vi "NM GlobalTest.vi"() -> ()   [LabVIEW 2010] (continued)
                        }
                        frame "DAQmx" {
                          n691 = call-poly <vilib>:"DAQmx Read.vi"("task/channels in"=w2908, "number of samples per channel"=w2904, "timeout"=w2905, "error in"=w2909) -> ("task out"=w2911:refnum<k21>, "data"=w2906:dbl[], "error out"=w2910:errorcluster)  [unwired: 9 in]
                        }
                      }
                      "data 37" <- w2890
                      "data 75" <- w2890
                    }
                    frame "sCnSWfm" {
                      n692 = case shown="\"DAQmx\"" w2914 {
                        tunnel: [w2927 w2935] -> w2921
                        tunnel: [w2928 w2932] -> w2920
                        tunnel: [w2929 w2937] -> w2915
                        tunnel: w2919 -> [w2925 w2933]
                        tunnel: w2918 -> [w2926 w2932]
                        tunnel: [w2924 w2936] -> w2917
                        tunnel: w2916 -> [w2924 w2934]
                        tunnel: w2913 -> [w2923 w2931]
                        tunnel: "samples per" -> [w2922 w2930]
                        frame "ULx", Default {
                          n693 = call-poly <vilib>:"ULx Read.vi"("task in"=w2926, "number of samples per channel"=w2922, "timeout"=w2923, "error in"=w2925) -> ("task out"=w2928:refnum<k24>, "data"=w2929:waveform(dbl), "error out"=w2927:errorcluster)  [unwired: 9 in]
                        }
                        frame "DAQmx" {
                          n694 = call-poly <vilib>:"DAQmx Read.vi"("task/channels in"=w2934, "number of samples per channel"=w2930, "timeout"=w2931, "error in"=w2933) -> ("task out"=w2936:refnum<k21>, "data"=w2937:waveform(dbl), "error out"=w2935:errorcluster)  [unwired: 9 in]
                        }
                      }
                      "data 38" <- w2915
                    }
                    frame "nCsSDbl" {
                      n695 = case shown="\"DAQmx\"" w2939 {
                        tunnel: [w2952 w2955] -> w2946
                        tunnel: [w2951 w2958] -> w2945
                        tunnel: [w2953 w2960] -> w2940
                        tunnel: w2944 -> [w2950 w2957]
                        tunnel: w2943 -> [w2949 w2955]
                        tunnel: [w2948 w2959] -> w2942
                        tunnel: w2941 -> [w2948 w2956]
                        tunnel: w2938 -> [w2947 w2954]
                        frame "ULx", Default {
                          n696 = call-poly <vilib>:"ULx Read.vi"("task in"=w2949, "timeout"=w2947, "error in"=w2950) -> ("task out"=w2952:refnum<k24>, "data"=w2953:dbl[], "error out"=w2951:errorcluster)  [unwired: 10 in]
                        }
                        frame "DAQmx" {
                          n697 = call-poly <vilib>:"DAQmx Read.vi"("task/channels in"=w2956, "timeout"=w2954, "error in"=w2957) -> ("task out"=w2959:refnum<k21>, "data"=w2960:dbl[], "error out"=w2958:errorcluster)  [unwired: 10 in]
                        }
                      }
                      "data 39" <- w2940
                    }
                    frame "nCsSWfm" {
                      n698 = case shown="\"DAQmx\"" w2962 {
                        tunnel: [w2975 w2978] -> w2969
                        tunnel: [w2974 w2981] -> w2968
                        tunnel: [w2976 w2983] -> w2963
                        tunnel: w2967 -> [w2972 w2980]
                        tunnel: w2966 -> [w2973 w2978]
                        tunnel: w2965 -> [w2971 w2979]
                        tunnel: [w2971 w2982] -> w2964
                        tunnel: w2961 -> [w2970 w2977]
                        frame "ULx", Default {
                          n699 = call-poly <vilib>:"ULx Read.vi"("task in"=w2973, "timeout"=w2970, "error in"=w2972) -> ("task out"=w2975:refnum<k24>, "data"=w2976:waveform(dbl)[], "error out"=w2974:errorcluster)  [unwired: 10 in]
                        }
                        frame "DAQmx" {
                          n700 = call-poly <vilib>:"DAQmx Read.vi"("task/channels in"=w2979, "timeout"=w2977, "error in"=w2980) -> ("task out"=w2982:refnum<k21>, "data"=w2983:waveform(dbl)[], "error out"=w2981:errorcluster)  [unwired: 10 in]
                        }
                      }
                      "data 40" <- w2963
                    }
                    frame "nCnS2D" {
                      n701 = case shown="\"DAQmx\"" w2986 {
                        tunnel: [w3000 w3004] -> w2993
                        tunnel: [w2999 w3008] -> w2992
                        tunnel: [w3001 w3009] -> w2987
                        tunnel: w2991 -> [w2997 w3006]
                        tunnel: w2990 -> [w2998 w3004]
                        tunnel: w2989 -> [w2996 w3005]
                        tunnel: [w2996 w3007] -> w2988
                        tunnel: w2985 -> [w2995 w3002]
                        tunnel: "samples per" -> [w2994 w3003]
                        frame "ULx", Default {
                          n702 = call-poly <vilib>:"ULx Read.vi"("task in"=w2998, "number of samples per channel"=w2994, "timeout"=w2995, "error in"=w2997) -> ("task out"=w3000:refnum<k24>, "data"=w3001:dbl[][], "error out"=w2999:errorcluster)  [unwired: 9 in]
                        }
                        frame "DAQmx" {
                          n703 = call-poly <vilib>:"DAQmx Read.vi"("task/channels in"=w3005, "number of samples per channel"=w3003, "timeout"=w3002, "error in"=w3006) -> ("task out"=w3007:refnum<k21>, "data"=w3009:dbl[][], "error out"=w3008:errorcluster)  [unwired: 9 in]
                        }
                      }
                      "data 41" <- w2987
                      "data 76" <- w2987
                    }
                    frame "nCnS1DWfm" {
                      n704 = case shown="\"DAQmx\"" w3012 {
                        tunnel: [w3025 w3033] -> w3019
                        tunnel: [w3026 w3030] -> w3018
                        tunnel: [w3027 w3035] -> w3013
                        tunnel: w3017 -> [w3023 w3031]
                        tunnel: w3016 -> [w3024 w3030]
                        tunnel: [w3022 w3034] -> w3015
                        tunnel: w3014 -> [w3022 w3032]
                        tunnel: w3011 -> [w3021 w3029]
                        tunnel: "samples per" -> [w3020 w3028]
                        frame "ULx", Default {
                          n705 = call-poly <vilib>:"ULx Read.vi"("task in"=w3024, "number of samples per channel"=w3020, "timeout"=w3021, "error in"=w3023) -> ("task out"=w3026:refnum<k24>, "data"=w3027:waveform(dbl)[], "error out"=w3025:errorcluster)  [unwired: 9 in]
                        }
                        frame "DAQmx" {
                          n706 = call-poly <vilib>:"DAQmx Read.vi"("task/channels in"=w3032, "number of samples per channel"=w3028, "timeout"=w3029, "error in"=w3031) -> ("task out"=w3034:refnum<k21>, "data"=w3035:waveform(dbl)[], "error out"=w3033:errorcluster)  [unwired: 9 in]
                        }
                      }
                      "data 42" <- w3013
                    }
                    frame "2DI16" {
                      n707 = case shown="\"DAQmx\"" w3038 {
                        tunnel: [w3048 w3055] -> w3041
                        tunnel: [_ w3056] -> w3040
                        tunnel: w3043 -> [w3048 w3053]
                        tunnel: w3044 -> [w3047 w3051]
                        tunnel: [w3046 w3054] -> w3042
                        tunnel: w3045 -> [w3046 w3052]
                        tunnel: [w3047 w3051] -> w3039
                        tunnel: "samples per" -> [_ w3050]
                        tunnel: w3036 -> [_ w3049]
                        frame "ULx", Default {
                        }
                        frame "DAQmx" {
                          n708 = call-poly <vilib>:"DAQmx Read.vi"("task/channels in"=w3052, "number of samples per channel"=w3050, "timeout"=w3049, "error in"=w3053) -> ("task out"=w3054:refnum<k21>, "data"=w3056:i16[][], "error out"=w3055:errorcluster)  [unwired: 9 in]
                        }
                      }
                      "data 43" <- w3040
                    }
                    frame "2DI32" {
                      n709 = case shown="\"DAQmx\"" w3058 {
                        tunnel: [w3069 w3076] -> w3062
                        tunnel: [_ w3077] -> w3060
                        tunnel: "samples per" -> [_ w3072]
                        tunnel: w3065 -> [w3069 w3074]
                        tunnel: w3064 -> [w3068 w3071]
                        tunnel: [w3067 w3075] -> w3061
                        tunnel: w3063 -> [w3067 w3073]
                        tunnel: [w3068 w3071] -> w3059
                        tunnel: w3057 -> [_ w3070]
                        frame "ULx", Default {
                        }
                        frame "DAQmx" {
                          n710 = call-poly <vilib>:"DAQmx Read.vi"("task/channels in"=w3073, "number of samples per channel"=w3072, "timeout"=w3070, "error in"=w3074) -> ("task out"=w3075:refnum<k21>, "data"=w3077:i32[][], "error out"=w3076:errorcluster)  [unwired: 9 in]
                        }
                      }
                      "data 44" <- w3060
                    }
                    frame "2DU16" {
                      n711 = case shown="\"DAQmx\"" w3079 {
                        tunnel: [w3090 w3097] -> w3083
                        tunnel: [_ w3098] -> w3081
                        tunnel: "samples per" -> [_ w3093]
                        tunnel: w3086 -> [w3090 w3095]
                        tunnel: w3085 -> [w3089 w3092]
                        tunnel: [w3088 w3096] -> w3082
                        tunnel: w3084 -> [w3088 w3094]
                        tunnel: [w3089 w3092] -> w3080
                        tunnel: w3078 -> [_ w3091]
                        frame "ULx", Default {
                        }
                        frame "DAQmx" {
                          n712 = call-poly <vilib>:"DAQmx Read.vi"("task/channels in"=w3094, "number of samples per channel"=w3093, "timeout"=w3091, "error in"=w3095) -> ("task out"=w3096:refnum<k21>, "data"=w3098:u16[][], "error out"=w3097:errorcluster)  [unwired: 9 in]
                        }
                      }
                      "data 45" <- w3081
                    }
                    frame "2DU32" {
                      n713 = case shown="\"DAQmx\"" w3100 {
                        tunnel: [w3111 w3118] -> w3104
                        tunnel: [_ w3119] -> w3102
                        tunnel: "samples per" -> [_ w3114]
                        tunnel: w3107 -> [w3111 w3116]
                        tunnel: w3106 -> [w3110 w3113]
                        tunnel: [w3109 w3117] -> w3103
                        tunnel: w3105 -> [w3109 w3115]
                        tunnel: [w3110 w3113] -> w3101
                        tunnel: w3099 -> [_ w3112]
                        frame "ULx", Default {
                        }
                        frame "DAQmx" {
                          n714 = call-poly <vilib>:"DAQmx Read.vi"("task/channels in"=w3115, "number of samples per channel"=w3114, "timeout"=w3112, "error in"=w3116) -> ("task out"=w3117:refnum<k21>, "data"=w3119:u32[][], "error out"=w3118:errorcluster)  [unwired: 9 in]
                        }
                      }
                      "data 46" <- w3102
                    }
                  }
                }
                frame "Digital" {
                  n715 = case shown="\" Single Channel\"" "nCOrsCDin" {
                    tunnel: w3127 -> [w3136 w3387]
                    tunnel: w3126 -> [w3135 w3386]
                    tunnel: w3125 -> [w3134 w3385]
                    tunnel: [w3130 w3381] -> w3122
                    tunnel: [w3131 w3382] -> w3123
                    tunnel: [w3132 w3383] -> w3124
                    tunnel: w3121 -> [w3133 w3384]
                    tunnel: w3120 -> [w3129 w3380]
                    frame "Multi-Channel", Default {
                      n716 = case shown="\"nCsSWv\"" "nCDIn" {
                        tunnel: [w3145 w3169 w3191 w3215 w3237 w3260 w3284 w3311 w3336 w3362] -> w3132
                        tunnel: [w3146 w3168 w3192 w3214 w3238 w3261 w3285 w3310 w3337 w3361] -> w3131
                        tunnel: w3133 -> [w3143 w3165 w3189 w3212 w3234 w3259 w3282 w3308 w3334 w3360]
                        tunnel: w3135 -> [w3141 w3166 w3187 w3210 w3233 w3257 w3280 w3306 w3333 w3359]
                        tunnel: w3136 -> [w3142 w3163 w3185 w3208 w3231 w3256 w3279 w3304 w3330 w3358]
                        tunnel: w3134 -> [w3140 w3164 w3188 w3211 w3235 w3258 w3281 w3307 w3332 w3357]
                        tunnel: [w3139 w3162 w3186 w3209 w3232 w3255 w3278 w3305 w3331 w3356] -> w3130
                        tunnel: w3129 -> [w3138 w3161 w3184 w3207 w3230 w3254 w3277 w3303 w3329 w3355]
                        frame "nCsSBool", Default {
                          n717 = case shown="\"DAQmx\"" w3143 {
                            tunnel: [w3153 w3155] -> w3146
                            tunnel: [w3152 w3160] -> w3145
                            tunnel: [w3151 w3159] -> w3144
                            tunnel: w3142 -> [w3148 w3158]
                            tunnel: w3141 -> [w3150 w3155]
                            tunnel: w3140 -> [w3149 w3157]
                            tunnel: [w3148 w3156] -> w3139
                            tunnel: w3138 -> [w3147 w3154]
                            frame "ULx", Default {
                              n718 = call-poly <vilib>:"ULx Read.vi"("task in"=w3150, "timeout"=w3147, "error in"=w3149) -> ("task out"=w3153:refnum<k24>, "data"=w3151:bool[], "error out"=w3152:errorcluster)  [unwired: 10 in]
                            }
                            frame "DAQmx" {
                              n719 = call-poly <vilib>:"DAQmx Read.vi"("task/channels in"=w3158, "timeout"=w3154, "error in"=w3157) -> ("task out"=w3156:refnum<k21>, "data"=w3159:bool[], "error out"=w3160:errorcluster)  [unwired: 10 in]
                            }
                          }
                          "data 47" <- w3144
                        }
                        frame "nCsS2D" {
                          n720 = case shown="\"DAQmx\"" w3165 {
                            tunnel: [w3176 w3183] -> w3169
                            tunnel: [w3175 w3178] -> w3168
                            tunnel: [w3174 w3179] -> w3167
                            tunnel: w3166 -> [w3173 w3178]
                            tunnel: w3164 -> [w3172 w3182]
                            tunnel: w3163 -> [w3171 w3181]
                            tunnel: [w3171 w3180] -> w3162
                            tunnel: w3161 -> [w3170 w3177]
                            frame "ULx", Default {
                              n721 = call-poly <vilib>:"ULx Read.vi"("task in"=w3173, "timeout"=w3170, "error in"=w3172) -> ("task out"=w3175:refnum<k24>, "data"=w3174:bool[][], "error out"=w3176:errorcluster)  [unwired: 10 in]
                            }
                            frame "DAQmx" {
                              n722 = call-poly <vilib>:"DAQmx Read.vi"("task/channels in"=w3181, "timeout"=w3177, "error in"=w3182) -> ("task out"=w3180:refnum<k21>, "data"=w3179:bool[][], "error out"=w3183:errorcluster)  [unwired: 10 in]
                            }
                          }
                          "data 48" <- w3167
                        }
                        frame "nCsSU8" {
                          n723 = case shown="\"DAQmx\"" w3189 {
                            tunnel: [w3199 w3201] -> w3192
                            tunnel: [w3198 w3205] -> w3191
                            tunnel: [w3197 w3204] -> w3190
                            tunnel: w3188 -> [w3196 w3206]
                            tunnel: w3187 -> [w3195 w3201]
                            tunnel: [w3194 w3203] -> w3186
                            tunnel: w3185 -> [w3194 w3202]
                            tunnel: w3184 -> [w3193 w3200]
                            frame "ULx", Default {
                              n724 = call-poly <vilib>:"ULx Read.vi"("task in"=w3195, "timeout"=w3193, "error in"=w3196) -> ("task out"=w3199:refnum<k24>, "data"=w3197:u8[], "error out"=w3198:errorcluster)  [unwired: 10 in]
                            }
                            frame "DAQmx" {
                              n725 = call-poly <vilib>:"DAQmx Read.vi"("task/channels in"=w3202, "timeout"=w3200, "error in"=w3206) -> ("task out"=w3203:refnum<k21>, "data"=w3204:u8[], "error out"=w3205:errorcluster)  [unwired: 10 in]
                            }
                          }
                          "data 49" <- w3190
                        }
                        frame "nCsSU16" {
                          n726 = case shown="\"DAQmx\"" w3212 {
                            tunnel: [w3222 w3228] -> w3215
                            tunnel: [w3221 w3224] -> w3214
                            tunnel: [w3220 w3227] -> w3213
                            tunnel: w3211 -> [w3219 w3229]
                            tunnel: w3210 -> [w3218 w3224]
                            tunnel: [w3217 w3226] -> w3209
                            tunnel: w3208 -> [w3217 w3225]
                            tunnel: w3207 -> [w3216 w3223]
                            frame "ULx", Default {
                              n727 = call-poly <vilib>:"ULx Read.vi"("task in"=w3218, "timeout"=w3216, "error in"=w3219) -> ("task out"=w3221:refnum<k24>, "data"=w3220:u16[], "error out"=w3222:errorcluster)  [unwired: 10 in]
                            }
                            frame "DAQmx" {
                              n728 = call-poly <vilib>:"DAQmx Read.vi"("task/channels in"=w3225, "timeout"=w3223, "error in"=w3229) -> ("task out"=w3226:refnum<k21>, "data"=w3227:u16[], "error out"=w3228:errorcluster)  [unwired: 10 in]
                            }
                          }
                          "data 50" <- w3213
                        }
                        frame "nCsSU32" {
                          n729 = case shown="\"DAQmx\"" w3234 {
                            tunnel: [w3245 w3247] -> w3238
                            tunnel: [w3244 w3250] -> w3237
                            tunnel: [w3243 w3252] -> w3236
                            tunnel: w3235 -> [w3242 w3249]
                            tunnel: w3233 -> [w3241 w3247]
                            tunnel: [w3240 w3251] -> w3232
                            tunnel: w3231 -> [w3240 w3248]
                            tunnel: w3230 -> [w3239 w3246]
                            frame "ULx", Default {
                              n730 = call-poly <vilib>:"ULx Read.vi"("task in"=w3241, "timeout"=w3239, "error in"=w3242) -> ("task out"=w3245:refnum<k24>, "data"=w3243:u32[], "error out"=w3244:errorcluster)  [unwired: 10 in]
                            }
                            frame "DAQmx" {
                              n731 = call-poly <vilib>:"DAQmx Read.vi"("task/channels in"=w3248, "timeout"=w3246, "error in"=w3249) -> ("task out"=w3251:refnum<k21>, "data"=w3252:u32[], "error out"=w3250:errorcluster)  [unwired: 10 in]
                            }
                          }
                          "data 51" <- w3236
                        }
                        frame "nCsSWv" {
                          n732 = case shown="\"ULx\", Default" w3259 {
                            tunnel: [w3268 w3270] -> w3261
                            tunnel: [w3267 w3274] -> w3260
                            tunnel: [w3266 w3275] -> w3253
                            tunnel: w3258 -> [w3265 w3273]
                            tunnel: w3257 -> [w3264 w3270]
                            tunnel: w3256 -> [w3263 w3272]
                            tunnel: [w3263 w3271] -> w3255
                            tunnel: w3254 -> [w3262 w3269]
                            frame "ULx", Default {
                              n733 = call-poly <vilib>:"ULx Read.vi"("task in"=w3264, "timeout"=w3262, "error in"=w3265) -> ("task out"=w3268:refnum<k24>, "data"=w3266:digitalwaveform[], "error out"=w3267:errorcluster)  [unwired: 10 in]
                            }
                            frame "DAQmx" {
                              n734 = call-poly <vilib>:"DAQmx Read.vi"("task/channels in"=w3272, "timeout"=w3269, "error in"=w3273) -> ("task out"=w3271:refnum<k21>, "data"=w3275:digitalwaveform[], "error out"=w3274:errorcluster)  [unwired: 10 in]
                            }
                          }
                          "data 52" <- w3253
                        }
                        frame "nCnSU8" {
                          n735 = case shown="\"ULx\", Default" w3282 {
                            tunnel: [w3293 w3296] -> w3285
                            tunnel: [w3292 w3300] -> w3284
                            tunnel: [w3291 w3301] -> w3283
                            tunnel: w3281 -> [w3290 w3299]
                            tunnel: w3280 -> [w3289 w3296]
                            tunnel: w3279 -> [w3288 w3298]
                            tunnel: [w3288 w3297] -> w3278
                            tunnel: w3277 -> [w3287 w3295]
                            tunnel: "samples per" -> [w3286 w3294]
                            frame "ULx", Default {
                              n736 = call-poly <vilib>:"ULx Read.vi"("task in"=w3289, "number of samples per channel"=w3286, "timeout"=w3287, "error in"=w3290) -> ("task out"=w3293:refnum<k24>, "data"=w3291:u8[][], "error out"=w3292:errorcluster)  [unwired: 9 in]
                            }
                            frame "DAQmx" {
                              n737 = call-poly <vilib>:"DAQmx Read.vi"("task/channels in"=w3298, "number of samples per channel"=w3294, "timeout"=w3295, "error in"=w3299) -> ("task out"=w3297:refnum<k21>, "data"=w3301:u8[][], "error out"=w3300:errorcluster)  [unwired: 9 in]
                            }
                          }
                          "data 53" <- w3283
                        }
                        frame "nCnSU16" {
                          n738 = case shown="\"DAQmx\"" w3308 {
                            tunnel: [w3319 w3326] -> w3311
                            tunnel: [w3318 w3322] -> w3310
                            tunnel: [w3317 w3327] -> w3309
                            tunnel: w3307 -> [w3316 w3324]
                            tunnel: w3306 -> [w3315 w3322]
                            tunnel: [w3314 w3325] -> w3305
                            tunnel: w3304 -> [w3314 w3323]
                            tunnel: w3303 -> [w3313 w3320]
                            tunnel: "samples per" -> [w3312 w3321]
                            frame "ULx", Default {
                              n739 = call-poly <vilib>:"ULx Read.vi"("task in"=w3315, "number of samples per channel"=w3312, "timeout"=w3313, "error in"=w3316) -> ("task out"=w3318:refnum<k24>, "data"=w3317:u16[][], "error out"=w3319:errorcluster)  [unwired: 9 in]
                            }
                            frame "DAQmx" {
                              n740 = call-poly <vilib>:"DAQmx Read.vi"("task/channels in"=w3323, "number of samples per channel"=w3321, "timeout"=w3320, "error in"=w3324) -> ("task out"=w3325:refnum<k21>, "data"=w3327:u16[][], "error out"=w3326:errorcluster)  [unwired: 9 in]
                            }
                          }
                          "data 54" <- w3309
                        }
                        frame "nCnSU32" {
                          n741 = case shown="\"DAQmx\"" w3334 {
                            tunnel: [w3345 w3348] -> w3337
                            tunnel: [w3344 w3351] -> w3336
                            tunnel: [w3343 w3353] -> w3335
                            tunnel: w3333 -> [w3342 w3348]
                            tunnel: w3332 -> [w3341 w3350]
                            tunnel: [w3340 w3352] -> w3331
                            tunnel: w3330 -> [w3340 w3349]
                            tunnel: w3329 -> [w3339 w3346]
                            tunnel: "samples per" -> [w3338 w3347]
                            frame "ULx", Default {
                              n742 = call-poly <vilib>:"ULx Read.vi"("task in"=w3342, "number of samples per channel"=w3338, "timeout"=w3339, "error in"=w3341) -> ("task out"=w3345:refnum<k24>, "data"=w3343:u32[][], "error out"=w3344:errorcluster)  [unwired: 9 in]
                            }
                            frame "DAQmx" {
                              n743 = call-poly <vilib>:"DAQmx Read.vi"("task/channels in"=w3349, "number of samples per channel"=w3347, "timeout"=w3346, "error in"=w3350) -> ("task out"=w3352:refnum<k21>, "data"=w3353:u32[][], "error out"=w3351:errorcluster)  [unwired: 9 in]
                            }
                          }
                          "data 55" <- w3335
                        }
                        frame "nCnSWv" {
                          n744 = case shown="\"ULx\", Default" w3360 {
                            tunnel: [w3371 w3379] -> w3363
                            tunnel: [w3370 w3378] -> w3362
                            tunnel: [w3369 w3374] -> w3361
                            tunnel: w3359 -> [w3368 w3374]
                            tunnel: w3358 -> [w3366 w3377]
                            tunnel: w3357 -> [w3367 w3376]
                            tunnel: [w3366 w3375] -> w3356
                            tunnel: w3355 -> [w3365 w3372]
                            tunnel: "samples per" -> [w3364 w3373]
                            frame "ULx", Default {
                              n745 = call-poly <vilib>:"ULx Read.vi"("task in"=w3368, "number of samples per channel"=w3364, "timeout"=w3365, "error in"=w3367) -> ("task out"=w3369:refnum<k24>, "data"=w3371:digitalwaveform[], "error out"=w3370:errorcluster)  [unwired: 9 in]
                            }
                            frame "DAQmx" {
                              n746 = call-poly <vilib>:"DAQmx Read.vi"("task/channels in"=w3377, "number of samples per channel"=w3373, "timeout"=w3372, "error in"=w3376) -> ("task out"=w3375:refnum<k21>, "data"=w3379:digitalwaveform[], "error out"=w3378:errorcluster)  [unwired: 9 in]
                            }
                          }
                          "data 56" <- w3363
                        }
                      }
                    }
                    frame " Single Channel" {
                      n747 = case shown="\"sCnSU8\"" "sCDin" {
                        tunnel: [w3396 w3420 w3442 w3466 w3488 w3511 w3535 w3562 w3587 w3614] -> w3383
                        tunnel: [w3397 w3419 w3443 w3465 w3489 w3512 w3536 w3561 w3588 w3613] -> w3382
                        tunnel: w3384 -> [w3395 w3417 w3441 w3464 w3486 w3510 w3533 w3560 w3585 w3611]
                        tunnel: w3386 -> [w3393 w3418 w3439 w3462 w3485 w3508 w3531 w3558 w3584 w3610]
                        tunnel: w3387 -> [w3394 w3415 w3437 w3460 w3483 w3507 w3530 w3556 w3581 w3609]
                        tunnel: w3385 -> [w3392 w3416 w3440 w3463 w3487 w3509 w3532 w3559 w3583 w3608]
                        tunnel: [w3391 w3414 w3438 w3461 w3484 w3506 w3529 w3557 w3582 w3607] -> w3381
                        tunnel: w3380 -> [w3389 w3412 w3435 w3458 w3481 w3504 w3527 w3554 w3579 w3605]
                        frame "sCsSBool", Default {
                          n748 = case shown="\"ULx\", Default" w3395 {
                            tunnel: [w3404 w3406] -> w3397
                            tunnel: [w3403 w3411] -> w3396
                            tunnel: w3394 -> [w3399 w3410]
                            tunnel: w3393 -> [w3402 w3406]
                            tunnel: w3392 -> [w3401 w3409]
                            tunnel: [w3399 w3408] -> w3391
                            tunnel: [w3400 w3407] -> w3390
                            tunnel: w3389 -> [w3398 w3405]
                            frame "ULx", Default {
                              n749 = call-poly <vilib>:"ULx Read.vi"("task in"=w3402, "timeout"=w3398, "error in"=w3401) -> ("task out"=w3404:refnum<k24>, "data"=w3400:bool, "error out"=w3403:errorcluster)  [unwired: 10 in]
                            }
                            frame "DAQmx" {
                              n750 = call-poly <vilib>:"DAQmx Read.vi"("task/channels in"=w3410, "timeout"=w3405, "error in"=w3409) -> ("task out"=w3408:refnum<k21>, "data"=w3407:bool, "error out"=w3411:errorcluster)  [unwired: 10 in]
                            }
                          }
                          "data 57" <- w3390
                        }
                        frame "sCsS1D" {
                          n751 = case shown="\"DAQmx\"" w3417 {
                            tunnel: [w3427 w3434] -> w3420
                            tunnel: [w3426 w3429] -> w3419
                            tunnel: [w3425 w3430] -> w3413
                            tunnel: w3418 -> [w3424 w3429]
                            tunnel: w3416 -> [w3423 w3433]
                            tunnel: w3415 -> [w3422 w3432]
                            tunnel: [w3422 w3431] -> w3414
                            tunnel: w3412 -> [w3421 w3428]
                            frame "ULx", Default {
                              n752 = call-poly <vilib>:"ULx Read.vi"("task in"=w3424, "timeout"=w3421, "error in"=w3423) -> ("task out"=w3426:refnum<k24>, "data"=w3425:bool[], "error out"=w3427:errorcluster)  [unwired: 10 in]
                            }
                            frame "DAQmx" {
                              n753 = call-poly <vilib>:"DAQmx Read.vi"("task/channels in"=w3432, "timeout"=w3428, "error in"=w3433) -> ("task out"=w3431:refnum<k21>, "data"=w3430:bool[], "error out"=w3434:errorcluster)  [unwired: 10 in]
                            }
                          }
                          "data 58" <- w3413
                        }
                        frame "sCsSU8" {
                          n754 = case shown="\"DAQmx\"" w3441 {
                            tunnel: [w3450 w3452] -> w3443
                            tunnel: [w3449 w3456] -> w3442
                            tunnel: [w3448 w3455] -> w3436
                            tunnel: w3440 -> [w3447 w3457]
                            tunnel: w3439 -> [w3446 w3452]
                            tunnel: [w3445 w3454] -> w3438
                            tunnel: w3437 -> [w3445 w3453]
                            tunnel: w3435 -> [w3444 w3451]
                            frame "ULx", Default {
                              n755 = call-poly <vilib>:"ULx Read.vi"("task in"=w3446, "timeout"=w3444, "error in"=w3447) -> ("task out"=w3450:refnum<k24>, "data"=w3448:u8, "error out"=w3449:errorcluster)  [unwired: 10 in]
                            }
                            frame "DAQmx" {
                              n756 = call-poly <vilib>:"DAQmx Read.vi"("task/channels in"=w3453, "timeout"=w3451, "error in"=w3457) -> ("task out"=w3454:refnum<k21>, "data"=w3455:u8, "error out"=w3456:errorcluster)  [unwired: 10 in]
                            }
                          }
                          "data 59" <- w3436
                        }
                        frame "sCsSU16" {
                          n757 = case shown="\"DAQmx\"" w3464 {
                            tunnel: [w3473 w3479] -> w3466
                            tunnel: [w3472 w3475] -> w3465
                            tunnel: [w3471 w3478] -> w3459
                            tunnel: w3463 -> [w3470 w3480]
                            tunnel: w3462 -> [w3469 w3475]
                            tunnel: [w3468 w3477] -> w3461
                            tunnel: w3460 -> [w3468 w3476]
                            tunnel: w3458 -> [w3467 w3474]
                            frame "ULx", Default {
                              n758 = call-poly <vilib>:"ULx Read.vi"("task in"=w3469, "timeout"=w3467, "error in"=w3470) -> ("task out"=w3472:refnum<k24>, "data"=w3471:u16, "error out"=w3473:errorcluster)  [unwired: 10 in]
                            }
                            frame "DAQmx" {
                              n759 = call-poly <vilib>:"DAQmx Read.vi"("task/channels in"=w3476, "timeout"=w3474, "error in"=w3480) -> ("task out"=w3477:refnum<k21>, "data"=w3478:u16, "error out"=w3479:errorcluster)  [unwired: 10 in]
                            }
                          }
                          "data 60" <- w3459
                        }
                        frame "sCsSU32" {
                          n760 = case shown="\"ULx\", Default" w3486 {
                            tunnel: [w3496 w3498] -> w3489
                            tunnel: [w3495 w3501] -> w3488
                            tunnel: [w3494 w3503] -> w3482
                            tunnel: w3487 -> [w3493 w3500]
                            tunnel: w3485 -> [w3492 w3498]
                            tunnel: [w3491 w3502] -> w3484
                            tunnel: w3483 -> [w3491 w3499]
                            tunnel: w3481 -> [w3490 w3497]
                            frame "ULx", Default {
                              n761 = call-poly <vilib>:"ULx Read.vi"("task in"=w3492, "timeout"=w3490, "error in"=w3493) -> ("task out"=w3496:refnum<k24>, "data"=w3494:u32, "error out"=w3495:errorcluster)  [unwired: 10 in]
                            }
                            frame "DAQmx" {
                              n762 = call-poly <vilib>:"DAQmx Read.vi"("task/channels in"=w3499, "timeout"=w3497, "error in"=w3500) -> ("task out"=w3502:refnum<k21>, "data"=w3503:u32, "error out"=w3501:errorcluster)  [unwired: 10 in]
                            }
                          }
                          "data 61" <- w3482
                        }
                        frame "sCsSWv" {
                          n763 = case shown="\"DAQmx\"" w3510 {
                            tunnel: [w3519 w3521] -> w3512
                            tunnel: [w3518 w3525] -> w3511
                            tunnel: [w3517 w3526] -> w3505
                            tunnel: w3509 -> [w3516 w3524]
                            tunnel: w3508 -> [w3515 w3521]
                            tunnel: w3507 -> [w3514 w3523]
                            tunnel: [w3514 w3522] -> w3506
                            tunnel: w3504 -> [w3513 w3520]
                            frame "ULx", Default {
                              n764 = call-poly <vilib>:"ULx Read.vi"("task in"=w3515, "timeout"=w3513, "error in"=w3516) -> ("task out"=w3519:refnum<k24>, "data"=w3517:digitalwaveform, "error out"=w3518:errorcluster)  [unwired: 10 in]
                            }
                            frame "DAQmx" {
                              n765 = call-poly <vilib>:"DAQmx Read.vi"("task/channels in"=w3523, "timeout"=w3520, "error in"=w3524) -> ("task out"=w3522:refnum<k21>, "data"=w3526:digitalwaveform, "error out"=w3525:errorcluster)  [unwired: 10 in]
                            }
                          }
                          "data 62" <- w3505
                        }
                        frame "sCnSU8" {
                          n766 = case shown="\"ULx\", Default" w3533 {
                            tunnel: [w3544 w3546] -> w3536
                            tunnel: [w3543 w3551] -> w3535
                            tunnel: [w3542 w3552] -> w3528
                            tunnel: "samples per" -> [w3541 w3549]
                            tunnel: w3532 -> [w3540 w3550]
                            tunnel: w3531 -> [w3539 w3546]
                            tunnel: w3530 -> [w3538 w3548]
                            tunnel: [w3538 w3547] -> w3529
                            tunnel: w3527 -> [w3537 w3545]
                            frame "ULx", Default {
                              n767 = call-poly <vilib>:"ULx Read.vi"("task in"=w3539, "number of samples per channel"=w3541, "timeout"=w3537, "error in"=w3540) -> ("task out"=w3544:refnum<k24>, "data"=w3542:u8[], "error out"=w3543:errorcluster)  [unwired: 9 in]
                            }
                            frame "DAQmx" {
                              n768 = call-poly <vilib>:"DAQmx Read.vi"("task/channels in"=w3548, "number of samples per channel"=w3549, "timeout"=w3545, "error in"=w3550) -> ("task out"=w3547:refnum<k21>, "data"=w3552:u8[], "error out"=w3551:errorcluster)  [unwired: 9 in]
                            }
                          }
                          "data 63" <- w3528
                          "data 79" <- w3528
                        }
                        frame "sCnSU16" {
                          n769 = case shown="\"ULx\", Default" w3560 {
                            tunnel: [w3570 w3577] -> w3562
                            tunnel: [w3569 w3573] -> w3561
                            tunnel: [w3568 w3578] -> w3555
                            tunnel: w3559 -> [w3567 w3575]
                            tunnel: w3558 -> [w3566 w3573]
                            tunnel: [w3565 w3576] -> w3557
                            tunnel: w3556 -> [w3565 w3574]
                            tunnel: w3554 -> [w3564 w3572]
                            tunnel: "samples per" -> [w3563 w3571]
                            frame "ULx", Default {
                              n770 = call-poly <vilib>:"ULx Read.vi"("task in"=w3566, "number of samples per channel"=w3563, "timeout"=w3564, "error in"=w3567) -> ("task out"=w3569:refnum<k24>, "data"=w3568:u16[], "error out"=w3570:errorcluster)  [unwired: 9 in]
                            }
                            frame "DAQmx" {
                              n771 = call-poly <vilib>:"DAQmx Read.vi"("task/channels in"=w3574, "number of samples per channel"=w3571, "timeout"=w3572, "error in"=w3575) -> ("task out"=w3576:refnum<k21>, "data"=w3578:u16[], "error out"=w3577:errorcluster)  [unwired: 9 in]
                            }
                          }
                          "data 64" <- w3555
                          "data 77" <- w3555
                        }
                        frame "sCnSU32" {
                          n772 = case shown="\"ULx\", Default" w3585 {
                            tunnel: [w3596 w3598] -> w3588
                            tunnel: [w3595 w3602] -> w3587
                            tunnel: [w3594 w3604] -> w3580
                            tunnel: "samples per" -> [w3593 w3600]
                            tunnel: w3584 -> [w3592 w3598]
                            tunnel: w3583 -> [w3591 w3601]
                            tunnel: [w3590 w3603] -> w3582
                            tunnel: w3581 -> [w3590 w3599]
                            tunnel: w3579 -> [w3589 w3597]
                            frame "ULx", Default {
                              n773 = call-poly <vilib>:"ULx Read.vi"("task in"=w3592, "number of samples per channel"=w3593, "timeout"=w3589, "error in"=w3591) -> ("task out"=w3596:refnum<k24>, "data"=w3594:u32[], "error out"=w3595:errorcluster)  [unwired: 9 in]
                            }
                            frame "DAQmx" {
                              n774 = call-poly <vilib>:"DAQmx Read.vi"("task/channels in"=w3599, "number of samples per channel"=w3600, "timeout"=w3597, "error in"=w3601) -> ("task out"=w3603:refnum<k21>, "data"=w3604:u32[], "error out"=w3602:errorcluster)  [unwired: 9 in]
                            }
                          }
                          "data 65" <- w3580
                          "data 78" <- w3580
                        }
                        frame "sCnSWv" {
                          n775 = case shown="\"ULx\", Default" w3611 {
                            tunnel: [w3622 w3630] -> w3606
                            tunnel: [w3621 w3629] -> w3614
                            tunnel: [w3620 w3624] -> w3613
                            tunnel: "samples per" -> [w3619 w3627]
                            tunnel: w3610 -> [w3618 w3624]
                            tunnel: w3609 -> [w3616 w3628]
                            tunnel: w3608 -> [w3617 w3626]
                            tunnel: [w3616 w3625] -> w3607
                            tunnel: w3605 -> [w3615 w3623]
                            frame "ULx", Default {
                              n776 = call-poly <vilib>:"ULx Read.vi"("task in"=w3618, "number of samples per channel"=w3619, "timeout"=w3615, "error in"=w3617) -> ("task out"=w3620:refnum<k24>, "data"=w3622:digitalwaveform, "error out"=w3621:errorcluster)  [unwired: 9 in]
                            }
                            frame "DAQmx" {
                              n777 = call-poly <vilib>:"DAQmx Read.vi"("task/channels in"=w3628, "number of samples per channel"=w3627, "timeout"=w3623, "error in"=w3626) -> ("task out"=w3625:refnum<k21>, "data"=w3630:digitalwaveform, "error out"=w3629:errorcluster)  [unwired: 9 in]
                            }
                          }
                          "data 66" <- w3606
                        }
                      }
                    }
                  }
                }
                frame "Counter" {
                  n778 = case shown="\"nCnSDbl\"" "CtrRead" {
                    tunnel: w3637 -> [w3648 w3671 w3695 w3721 w3747 w3770 w3794 w3819]
                    tunnel: w3638 -> [w3647 w3670 w3694 w3720 w3746 w3769 w3793 w3818]
                    tunnel: [w3645 w3669 w3693 w3719 w3745 w3768 w3792 w3817] -> w3633
                    tunnel: [w3644 w3668 w3692 w3718 w3744 w3767 w3791 w3816] -> w3634
                    tunnel: w3636 -> [w3643 w3666 w3689 w3714 w3741 w3764 w3787 w3812]
                    tunnel: [w3642 w3665 w3688 w3715 w3740 w3763 w3786 w3811] -> w3635
                    tunnel: w3632 -> [w3641 w3664 w3687 w3713 w3739 w3762 w3785 w3810]
                    tunnel: w3631 -> [w3640 w3663 w3686 w3712 w3738 w3761 w3784 w3809]
                    frame "sCsSDbl", Default {
                      n779 = case shown="\"DAQmx\"" w3641 {
                        tunnel: w3648 -> [w3655 w3657]
                        tunnel: w3647 -> [w3654 w3661]
                        tunnel: [w3653 w3659] -> w3646
                        tunnel: [w3652 w3660] -> w3645
                        tunnel: [w3651 w3657] -> w3644
                        tunnel: w3643 -> [w3650 w3662]
                        tunnel: [w3650 w3658] -> w3642
                        tunnel: w3640 -> [w3649 w3656]
                        frame "ULx", Default {
                          n780 = call-poly <vilib>:"ULx Read.vi"("task in"=w3655, "timeout"=w3649, "error in"=w3654) -> ("task out"=w3651:refnum<k24>, "data"=w3653:dbl, "error out"=w3652:errorcluster)  [unwired: 10 in]
                        }
                        frame "DAQmx" {
                          n781 = call-poly <vilib>:"DAQmx Read.vi"("task/channels in"=w3662, "timeout"=w3656, "error in"=w3661) -> ("task out"=w3658:refnum<k21>, "data"=w3659:dbl, "error out"=w3660:errorcluster)  [unwired: 10 in]
                        }
                      }
                      "data 67" <- w3646
                    }
                    frame "sCsSU32" {
                      n782 = case shown="\"ULx\", Default" w3664 {
                        tunnel: w3671 -> [w3678 w3680]
                        tunnel: w3670 -> [w3677 w3685]
                        tunnel: [w3676 w3684] -> w3669
                        tunnel: [w3675 w3680] -> w3668
                        tunnel: [w3674 w3683] -> w3667
                        tunnel: w3666 -> [w3673 w3682]
                        tunnel: [w3673 w3681] -> w3665
                        tunnel: w3663 -> [w3672 w3679]
                        frame "ULx", Default {
                          n783 = call-poly <vilib>:"ULx Read.vi"("task in"=w3678, "timeout"=w3672, "error in"=w3677) -> ("task out"=w3675:refnum<k24>, "data"=w3674:u32, "error out"=w3676:errorcluster)  [unwired: 10 in]
                        }
                        frame "DAQmx" {
                          n784 = call-poly <vilib>:"DAQmx Read.vi"("task/channels in"=w3682, "timeout"=w3679, "error in"=w3685) -> ("task out"=w3681:refnum<k21>, "data"=w3683:u32, "error out"=w3684:errorcluster)  [unwired: 10 in]
                        }
                      }
                      "data 68" <- w3667
                    }
                    frame "sCnSDbl" {
                      n785 = case shown="\"ULx\", Default" w3687 {
                        tunnel: w3695 -> [w3703 w3705]
                        tunnel: w3694 -> [w3702 w3711]
                        tunnel: [w3701 w3710] -> w3693
                        tunnel: [w3700 w3705] -> w3692
                        tunnel: "samples per" -> [w3699 w3708]
                        tunnel: [w3698 w3709] -> w3690
                        tunnel: w3689 -> [w3697 w3707]
                        tunnel: [w3697 w3706] -> w3688
                        tunnel: w3686 -> [w3696 w3704]
                        frame "ULx", Default {
                          n786 = call-poly <vilib>:"ULx Read.vi"("task in"=w3703, "number of samples per channel"=w3699, "timeout"=w3696, "error in"=w3702) -> ("task out"=w3700:refnum<k24>, "data"=w3698:dbl[], "error out"=w3701:errorcluster)  [unwired: 9 in]
                        }
                        frame "DAQmx" {
                          n787 = call-poly <vilib>:"DAQmx Read.vi"("task/channels in"=w3707, "number of samples per channel"=w3708, "timeout"=w3704, "error in"=w3711) -> ("task out"=w3706:refnum<k21>, "data"=w3709:dbl[], "error out"=w3710:errorcluster)  [unwired: 9 in]
                        }
                      }
                      "data 69" <- w3690
                    }
                    frame "sCnSU32" {
                      n788 = case shown="\"DAQmx\"" w3713 {
                        tunnel: w3721 -> [w3729 w3731]
                        tunnel: w3720 -> [w3728 w3737]
                        tunnel: [w3727 w3736] -> w3719
                        tunnel: [w3726 w3731] -> w3718
                        tunnel: "samples per" -> [w3725 w3732]
                        tunnel: [w3724 w3734] -> w3716
                        tunnel: [w3723 w3735] -> w3715
                        tunnel: w3714 -> [w3723 w3733]
                        tunnel: w3712 -> [w3722 w3730]
                        frame "ULx", Default {
                          n789 = call-poly <vilib>:"ULx Read.vi"("task in"=w3729, "number of samples per channel"=w3725, "timeout"=w3722, "error in"=w3728) -> ("task out"=w3726:refnum<k24>, "data"=w3724:u32[], "error out"=w3727:errorcluster)  [unwired: 9 in]
                        }
                        frame "DAQmx" {
                          n790 = call-poly <vilib>:"DAQmx Read.vi"("task/channels in"=w3733, "number of samples per channel"=w3732, "timeout"=w3730, "error in"=w3737) -> ("task out"=w3735:refnum<k21>, "data"=w3734:u32[], "error out"=w3736:errorcluster)  [unwired: 9 in]
                        }
                      }
                      "data 70" <- w3716
                    }
                    frame "nCsSDbl" {
                      n791 = case shown="\"ULx\", Default" w3739 {
                        tunnel: w3747 -> [w3754 w3755]
                        tunnel: w3746 -> [w3753 w3759]
                        tunnel: [w3752 w3760] -> w3745
                        tunnel: [w3751 w3755] -> w3744
                        tunnel: [w3750 _] -> w3743
                        tunnel: "No equivalent NI function." -> [_ w3758]
                        tunnel: w3741 -> [w3749 w3756]
                        tunnel: [w3749 w3756] -> w3740
                        tunnel: w3738 -> [w3748 _]
                        frame "ULx", Default {
                          n792 = call-poly <vilib>:"ULx Read.vi"("task in"=w3754, "timeout"=w3748, "error in"=w3753) -> ("task out"=w3751:refnum<k24>, "data"=w3750:dbl[], "error out"=w3752:errorcluster)  [unwired: 10 in]
                        }
                        frame "DAQmx" {
                          n793 = call <vilib>:"Error Cluster From Error Code.vi"("error in (no error)"=w3759, "error message (\"\")"=w3758, "error code (0)"=5002) -> ("error out"=w3760:errorcluster)  [unwired: 6 in]
                        }
                      }
                      "data 71" <- w3743
                    }
                    frame "nCsSU32" {
                      n794 = case shown="\"DAQmx\"" w3762 {
                        tunnel: w3770 -> [w3777 w3778]
                        tunnel: w3769 -> [w3776 w3782]
                        tunnel: [w3775 w3781] -> w3768
                        tunnel: [w3774 w3778] -> w3767
                        tunnel: [w3773 _] -> w3766
                        tunnel: "No equivalent NI function." -> [_ w3780]
                        tunnel: w3764 -> [w3772 w3779]
                        tunnel: [w3772 w3779] -> w3763
                        tunnel: w3761 -> [w3771 _]
                        frame "ULx", Default {
                          n795 = call-poly <vilib>:"ULx Read.vi"("task in"=w3777, "timeout"=w3771, "error in"=w3776) -> ("task out"=w3774:refnum<k24>, "data"=w3773:u32[], "error out"=w3775:errorcluster)  [unwired: 10 in]
                        }
                        frame "DAQmx" {
                          n796 = call <vilib>:"Error Cluster From Error Code.vi"("error in (no error)"=w3782, "error message (\"\")"=w3780, "error code (0)"=5002) -> ("error out"=w3781:errorcluster)  [unwired: 6 in]
                        }
                      }
                      "data 72" <- w3766
                    }
                    frame "nCnSDbl" {
                      n797 = case shown="\"DAQmx\"" w3785 {
                        tunnel: w3794 -> [w3802 w3803]
                        tunnel: w3793 -> [w3801 w3806]
                        tunnel: [w3800 w3805] -> w3792
                        tunnel: [w3799 w3803] -> w3791
                        tunnel: "samples per" -> [w3798 _]
                        tunnel: [w3797 _] -> w3789
                        tunnel: "No equivalent NI function." -> [_ w3807]
                        tunnel: w3787 -> [w3796 w3804]
                        tunnel: [w3796 w3804] -> w3786
                        tunnel: w3784 -> [w3795 _]
                        frame "ULx", Default {
                          n798 = call-poly <vilib>:"ULx Read.vi"("task in"=w3802, "number of samples per channel"=w3798, "timeout"=w3795, "error in"=w3801) -> ("task out"=w3799:refnum<k24>, "data"=w3797:dbl[][], "error out"=w3800:errorcluster)  [unwired: 9 in]
                        }
                        frame "DAQmx" {
                          n799 = call <vilib>:"Error Cluster From Error Code.vi"("error in (no error)"=w3806, "error message (\"\")"=w3807, "error code (0)"=5002) -> ("error out"=w3805:errorcluster)  [unwired: 6 in]
                        }
                      }
                      "data 73" <- w3789
                    }
                    frame "nCnSU32" {
                      n800 = case shown="\"DAQmx\"" w3810 {
                        tunnel: w3819 -> [w3827 w3828]
                        tunnel: w3818 -> [w3826 w3832]
                        tunnel: [w3825 w3831] -> w3817
                        tunnel: [w3824 w3828] -> w3816
                        tunnel: "samples per" -> [w3823 _]
                        tunnel: [w3822 _] -> w3814
                        tunnel: "No equivalent NI function." -> [_ w3830]
                        tunnel: w3812 -> [w3821 w3829]
                        tunnel: [w3821 w3829] -> w3811
                        tunnel: w3809 -> [w3820 _]
                        frame "ULx", Default {
                          n801 = call-poly <vilib>:"ULx Read.vi"("task in"=w3827, "number of samples per channel"=w3823, "timeout"=w3820, "error in"=w3826) -> ("task out"=w3824:refnum<k24>, "data"=w3822:u32[][], "error out"=w3825:errorcluster)  [unwired: 9 in]
                        }
                        frame "DAQmx" {
                          n802 = call <vilib>:"Error Cluster From Error Code.vi"("error in (no error)"=w3832, "error message (\"\")"=w3830, "error code (0)"=5002) -> ("error out"=w3831:errorcluster)  [unwired: 6 in]
                        }
                      }
                      "data 74" <- w3814
                    }
                  }
                }
                frame "Composite" {
                  n803 = case shown="\"2D\", Default" "CompRd" {
                    tunnel: w3843 -> [w3855 w3877]
                    tunnel: w3842 -> [w3854 w3878]
                    tunnel: w3841 -> [w3853 w3879]
                    tunnel: [w3852 w3874] -> w3840
                    tunnel: [w3851 w3875] -> w3839
                    tunnel: [w3850 w3876] -> w3838
                    tunnel: w3837 -> [w3849 w3873]
                    tunnel: w3835 -> [w3846 w3870]
                    tunnel: "samples" -> [w3845 w3869]
                    frame "2D", Default {
                      n804 = case shown="\"ULx\", Default" w3849 {
                        tunnel: w3854 -> [w3865 w3868]
                        tunnel: w3855 -> [w3864 w3866]
                        tunnel: [w3863 w3866] -> w3850
                        tunnel: [w3862 w3868] -> w3851
                        tunnel: w3853 -> [w3861 w3867]
                        tunnel: [w3861 w3867] -> w3852
                        tunnel: [w3860 _] -> w3848
                        tunnel: [w3859 _] -> w3847
                        tunnel: w3846 -> [w3858 _]
                        tunnel: w3845 -> [w3857 _]
                        tunnel: [w3856 _] -> w3844
                        frame "ULx", Default {
                          n805 = call-poly <vilib>:"ULx Read.vi"("task in"=w3865, "number of samples per channel"=w3857, "timeout"=w3858, "error in"=w3864) -> ("task out"=w3862:refnum<k24>, "analog data"=w3860:dbl[][], "digital data"=w3859:u32[][], "counter data"=w3856:u32[][], "error out"=w3863:errorcluster)  [unwired: 7 in]
                        }
                        frame "DAQmx" {
                        }
                      }
                      "analog data 4" <- w3848
                      "digital data 3" <- w3847
                      "counter data" <- w3844
                    }
                    frame "1D Waveform" {
                      n806 = case shown="\"ULx\", Default" w3873 {
                        tunnel: w3878 -> [w3888 w3891]
                        tunnel: w3877 -> [w3887 w3889]
                        tunnel: [w3886 w3889] -> w3876
                        tunnel: [w3885 w3891] -> w3875
                        tunnel: w3879 -> [w3884 w3890]
                        tunnel: [w3884 w3890] -> w3874
                        tunnel: [w3883 _] -> w3872
                        tunnel: [w3882 _] -> w3871
                        tunnel: w3870 -> [w3881 _]
                        tunnel: w3869 -> [w3880 _]
                        frame "ULx", Default {
                          n807 = call-poly <vilib>:"ULx Read.vi"("task in"=w3888, "number of samples per channel"=w3880, "timeout"=w3881, "error in"=w3887) -> ("task out"=w3885:refnum<k24>, "analog data"=w3883:waveform(dbl)[], "digital data"=w3882:digitalwaveform[], "error out"=w3886:errorcluster)  [unwired: 7 in, 1 out]
                        }
                        frame "DAQmx" {
                        }
                      }
                      "analog data 3" <- w3872
                      "digital data 4" <- w3871
                    }
                  }
                }
              }
            }
          }
          n808 = case shown="True" "Once" {
            frame False {
            }
            frame True {
              n809 = local write "Read"(FALSE ("Read")) -> ()
            }
          }
          n810 = local write "Read"(w2807) -> ()
        }
        frame 12 {
          # "WAIT"
          n811 = flat-sequence {
            tunnel: w3897 -> [w3906]
            tunnel: w3901 -> [w3907]
            tunnel: w3902 -> [w3908]
            tunnel: w3903 -> [w3909]
            tunnel: [w3909] -> w3896
            tunnel: [w3908] -> w3895
            tunnel: [w3907] -> w3894
            tunnel: [w3906] -> w3893
            tunnel: w3892 -> [w3904]
            tunnel: [w3917] -> w3900
            tunnel: [w3916] -> w3899
            tunnel: [w3915] -> w3898
            tunnel: w3896 -> [w3920]
            tunnel: w3895 -> [w3919]
            tunnel: w3894 -> [w3918]
            tunnel: w3893 -> [w3914]
            frame #0 {
              n812 = for {
                N: 5 -> [_]
                tunnel: w3904 -> [w3910]
                n813 = Wait Until Next ms Multiple(millisecond multiple=w3910) -> ()  [unwired: 1 out]
                "Wait" <- TRUE
              }
            }
            frame #1 {
              n814 = case shown="\"ULx\", Default" w3914 {
                tunnel: w3919 -> [w3927 w3931]
                tunnel: w3920 -> [w3926 w3933]
                tunnel: [w3925 w3934] -> w3915
                tunnel: w3918 -> [w3924 w3932]
                tunnel: [w3924 w3930] -> w3917
                tunnel: [w3923 w3931] -> w3916
                tunnel: "timeout" -> [w3922 w3928]
                tunnel: [FALSE FALSE] -> w3912
                frame "ULx", Default {
                  n815 = call <vilib>:"ULx Wait Until Done.vi"("task in"=w3927, "timeout"=w3922, "error in"=w3926) -> ("task out"=w3923:refnum<k24>, "error out"=w3925:errorcluster)  [unwired: 11 in]
                }
                frame "DAQmx" {
                  n816 = call <vilib>:"DAQmx Wait Until Done.vi"("task/channels in"=w3932, "timeout (sec)"=w3928, "error in"=w3933) -> ("task out"=w3930:refnum<k21>, "error out"=w3934:errorcluster)  [unwired: 11 in]
                }
              }
              n817 = local write "Wait"(w3912) -> ()
            }
          }
        }
        frame 13 {
          # "Property Nodes"
          n818 = stacked-sequence {
            tunnel: w3943 -> [w3944 w3962]
            tunnel: w3942 -> [_ w3961]
            tunnel: w3941 -> [_ w3960]
            tunnel: w3940 -> [_ w3959]
